vi "image acquisition practice.vi"() -> ()   [LabVIEW 2014]
uses:
  <vilib>/vision/Image Controls.llb/IMAQ Image.ctl
  <vilib>/vision/NI_Vision_Development_Module.lvlib
panel:
  out "Selected Region of Interest":T1
  out "Image Out 2":T1(plugin-control)
  out "Image Out":T1(plugin-control)
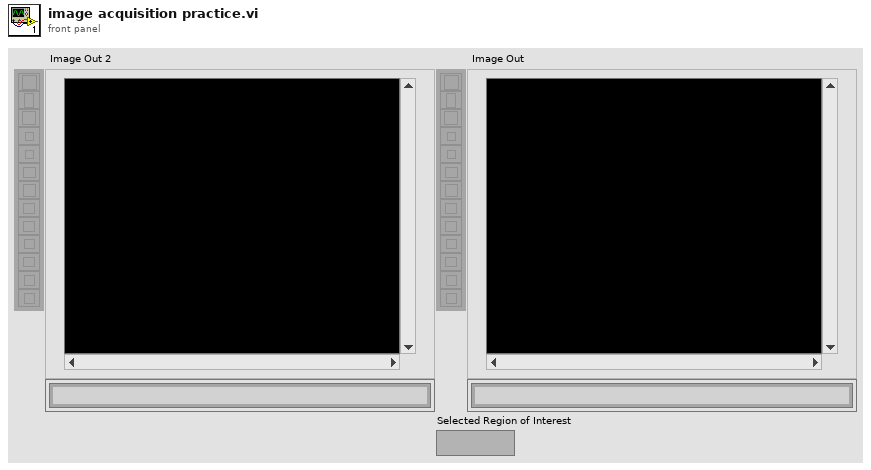
[diagram p1: front panel]
types:
  T1 = typedef "IMAQ Image.ctl" = refnum<image>
  T2 = typedef "ROI Descriptor" = cluster{"Global Rectangle":i32[], "Contours":cluster{"ID":enum32{"External", "Internal"}, "Type":u32, "Coordinates":i32[]}[]}
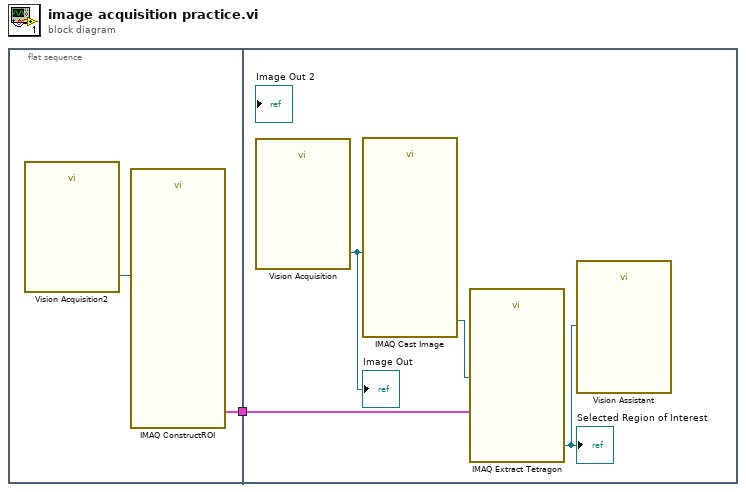
[diagram p0: block diagram]
diagram:
  n1 = flat-sequence {
    tunnel: [w2] -> w1
    tunnel: w1 -> [w4]
    frame #0 {
      n2 = call "Vision Acquisition2"() -> ("Image Out"=w3:T1)  [unwired: 26 in, 1 out]
      n3 = call "IMAQ ConstructROI"("Image"=w3) -> ("ROI Descriptor Out"=w2:T2)  [unwired: 7 in, 3 out]
    }
    frame #1 {
      n4 = call "Vision Acquisition"() -> ("Image Out"=w7:T1)  [unwired: 26 in, 1 out]
      "Image Out" <- w7
      n5 = call "IMAQ Cast Image"("Image Src"=w7) -> ("Image Dst Out"=w6:T1)  [unwired: 9 in, 1 out]
      n6 = call-poly "IMAQ Extract Tetragon"("ROI Descriptor"=w4, "Image Src"=w6) -> ("Image Dst Out"=w5:T1)  [unwired: 8 in, 1 out]
      "Selected Region of Interest" <- w5
      n7 = call "Vision Assistant"("Image In"=w5) -> ()  [unwired: 25 in, 2 out]
    }
  }
